vi "BMonitor.vi"   [LabVIEW 2016]
uses:
  Instrument_Setup.vi
  Global/Global Variables/Data_Display_global.vi
types:
  T1 = typedef "PSIO.ctl" = cluster{"Address":T2, "Version":enum16{"PS", "IPS"}}
  T2 = typedef "OxfordAddress.ctl" = cluster{"Com Port":i32, "ISOBUS Address":i32, "GPIB Address":i16, "Communication":enum16{"RS232", "ISOBUS", "GPIB", "Gateway"}}
  T3 = cluster{"Value":i16, "At rest":bool, "Sweeping":bool, "Rate limiting":bool}
  T4 = cluster{"Value":i16, "Hold":bool, "To set point":bool, "To zero":bool, "Clamped":bool}
  T5 = cluster{"Value":i16, "Off (at zero field)":bool, "On":bool, "Off (at field)":bool, "No switch fitted":bool, "Confirm":bool}
  T6 = cluster{"Value":i16, "Desired":u16, "Magnet":u16, "Commanded":u16, "Actual":u16}
  T7 = cluster{"Value":i16, "Quenched":bool, "Over heated":bool, "Warming up":bool}
  T8 = cluster{"Clamp":bool, "Settings":bool, "Switch Heater":bool, "Go to Zero":bool, "Go to set\nGo to Set":bool, "Go to Hold":bool, "Clamped":bool, "Quenched":bool, "Rate limit":bool, "Persistent":bool, "Hold":bool, "Set":bool, "Zero":bool, "Magnet (T)":dbl, "Leads (T)":dbl, "Magnet T (K)":dbl, "Confirm":bool, "Select":bool}
  T9 = typedef "PSSetupArray.ctl" = T10[]
  T10 = typedef "PSSetup.ctl" = cluster{"Max Sweep(4.2K)":dbl[unit], "Max Sweep(2.2K)":dbl[unit], "Switch htr dly":dbl[unit], "O/P contactor?":bool, "Max Field(4.2K)":dbl[unit], "Max Field(2.2K)":dbl[unit], "Description\n":string, "Settings.vi":path, "Max lead res":dbl[unit], "IO Info":T1, "Adjust shims":bool}
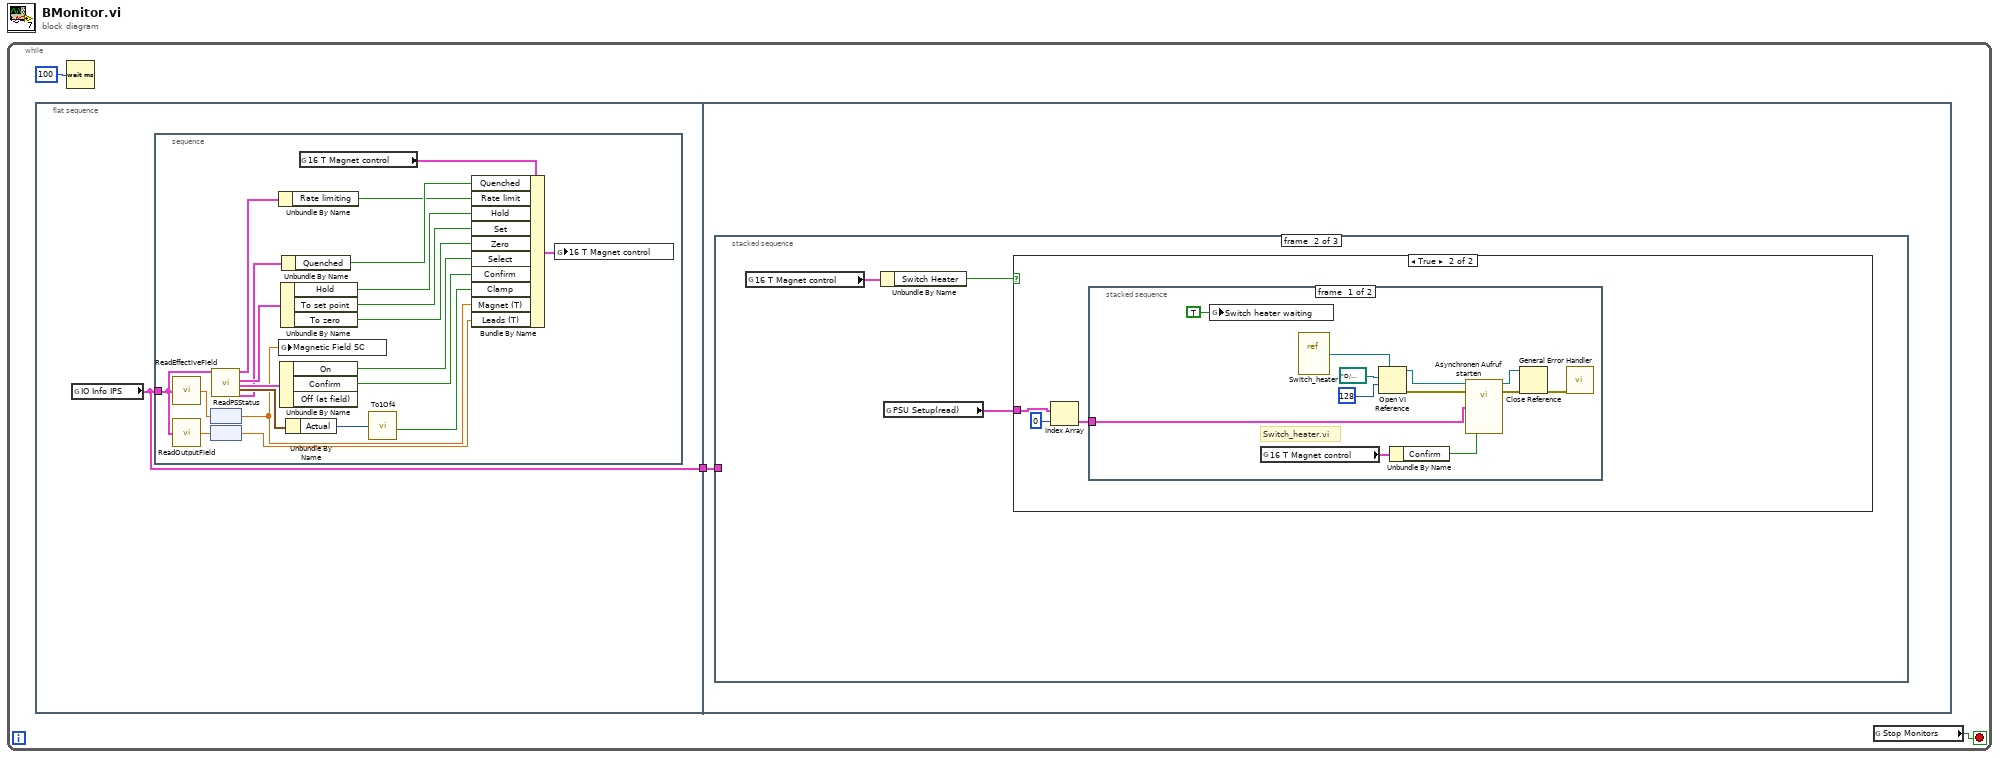
[diagram p0: block diagram]
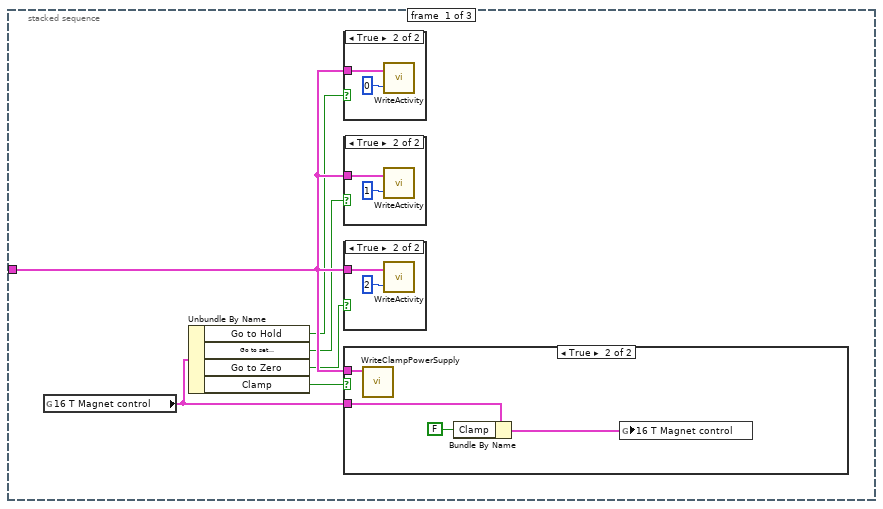
[diagram p2: hidden frame]
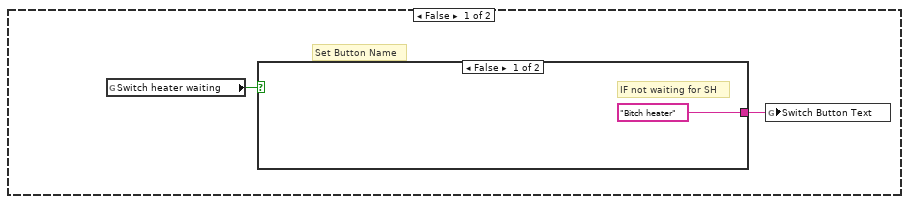
[diagram p7: hidden frame]
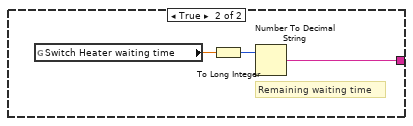
[diagram p8: hidden frame]
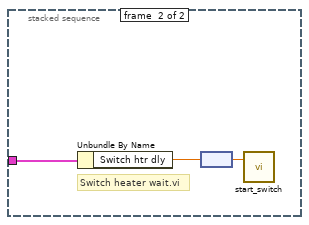
[diagram p9: hidden frame]
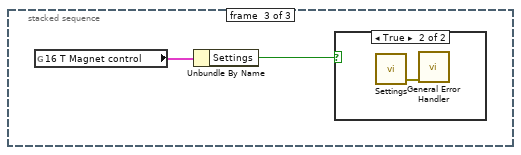
[diagram p10: hidden frame]
diagram:
  n1 = while {
    stop <- w3 stop-if-true
    n2 = flat-sequence {
      tunnel: [w4] -> w1
      tunnel: w1 -> [w26]
      frame #0 {
        n3 = global read "Instrument_Setup.vi" "IO Info IPS"() -> (w4:T1)
        n4 = stacked-sequence {
          tunnel: w4 -> [w7]
          frame #0 {
            n5 = call "ReadEffectiveField.vi"("IO Info"=w7) -> ("Effective field"=w6:dbl[unit])  [unwired: 2 out]
            n6 = call "ReadOutputField.vi"("IO Info"=w7) -> ("Field"=w9:dbl[unit])  [unwired: 2 out]
            n7 = node(w6) -> (w5:dbl)
            n8 = node(w9) -> (w8:dbl)
            n9 = call "ReadPSStatus.vi"("IO Info"=w7) -> ("Mode (n)"=w23:T3, "Activity"=w24:T4, "Switch Heater"=w22:T5, "Polarity"=w21:T6, "System Status (m)"=w20:T7)  [unwired: 10 in, 4 out]
            n10 = Unbundle By Name(w23) -> ("Rate limiting"=w15:bool)
            n11 = global write "Data_Display_global.vi" "Magnetic Field SC"(w5) -> ()
            n12 = Unbundle By Name(w22) -> ("On"=w11:bool, "Confirm"=w10:bool)  [unwired: 1 out]
            n13 = Unbundle By Name(w24) -> ("Hold"=w14:bool, "To set point"=w13:bool, "To zero"=w12:bool)
            n14 = Unbundle By Name(w20) -> ("Quenched"=w16:bool)
            n15 = Unbundle By Name(w21) -> ("Actual"=w25:u16)
            n16 = global read "Data_Display_global.vi" "16 T Magnet control"() -> (w19:T8)
            n17 = call "To1Of4.vi"("Input"=w25) -> ("3"=w17:bool)  [unwired: 3 out]
            n18 = Bundle By Name(cluster=w19, "Quenched"=w16, "Rate limit"=w15, "Hold"=w14, "Set"=w13, "Zero"=w12, "Select"=w11, "Confirm"=w10, "Clamp"=w17, "Magnet (T)"=w5, "Leads (T)"=w8) -> (w18:T8)
            n19 = global write "Data_Display_global.vi" "16 T Magnet control"(w18) -> ()
          }
        }
      }
      frame #1 {
        n20 = stacked-sequence {
          tunnel: w26 -> [w32 _ _]
          frame #0 {
            n21 = global read "Data_Display_global.vi" "16 T Magnet control"() -> (w27:T8)
            n22 = Unbundle By Name(w27) -> ("Go to Hold"=w31:bool, "Go to set\nGo to Set"=w30:bool, "Go to Zero"=w29:bool, "Clamp"=w28:bool)
            n23 = case shown="True" w31 {
              tunnel: w32 -> [_ w42]
              frame False {
              }
              frame True {
                n24 = call "WriteActivity.vi"("Activity"=0, "IO Info"=w42) -> ()  [unwired: 1 in, 1 out]
              }
            }
            n25 = case shown="True" w30 {
              tunnel: w32 -> [_ w40]
              frame False {
              }
              frame True {
                n26 = call "WriteActivity.vi"("Activity"=1, "IO Info"=w40) -> ()  [unwired: 1 in, 1 out]
              }
            }
            n27 = case shown="True" w29 {
              tunnel: w32 -> [_ w38]
              frame False {
              }
              frame True {
                n28 = call "WriteActivity.vi"("Activity"=2, "IO Info"=w38) -> ()  [unwired: 1 in, 1 out]
              }
            }
            n29 = case shown="True" w28 {
              tunnel: w32 -> [_ w36]
              tunnel: w27 -> [_ w34]
              frame False {
              }
              frame True {
                n30 = call "WriteClampPowerSupply.vi"("IO Info"=w36) -> ()  [unwired: 9 in, 2 out]
                n31 = Bundle By Name(cluster=w34, "Clamp"=FALSE) -> (w33:T8)
                n32 = global write "Data_Display_global.vi" "16 T Magnet control"(w33) -> ()
              }
            }
          }
          frame #1 {
            n33 = global read "Data_Display_global.vi" "16 T Magnet control"() -> (w45:T8)
            n34 = Unbundle By Name(w45) -> ("Switch Heater"=w44:bool)
            n35 = global read "Instrument_Setup.vi" "PSU Setup(read)"() -> (w43:T9)
            n36 = case shown="True" w44 {
              tunnel: w43 -> [_ w54]
              frame False {
                # "Set Button Name"
                n37 = global read "Data_Display_global.vi" "Switch heater waiting"() -> (w47:bool)
                n38 = case shown="False" w47 {
                  tunnel: ["Bitch heater" w49] -> w46
                  frame False {
                    # "IF not waiting for SH"
                  }
                  frame True {
                    # "Remaining waiting time"
                    n39 = global read "Data_Display_global.vi" "Switch Heater waiting time"() -> (w51:dbl)
                    n40 = To Long Integer(number=w51) -> (32bit integer=w50:i32)
                    n41 = Number To Decimal String(number=w50) -> (decimal integer string=w49:string)  [unwired: 1 in]
                  }
                }
                n42 = global write "Data_Display_global.vi" "Switch Button Text"(w46) -> ()
              }
              frame True {
                n43 = Index Array(array=w54, index=0) -> (element=w52:T10)
                n44 = stacked-sequence {
                  tunnel: w52 -> [w55 w67]
                  frame #0 {
                    # "Switch_heater.vi"
                    n45 = global write "Data_Display_global.vi" "Switch heater waiting"(TRUE) -> ()
                    n46 = global read "Data_Display_global.vi" "16 T Magnet control"() -> (w57:T8)
                    n47 = vi-ref "Switch_heater.vi"() -> (w66:refnum<vi>)
                    n48 = Open VI Reference(type specifier VI Refnum (for type only)=w66, vi path=path "D:/Cryostat Software/CryoTUM-V1.0/sub_vi-s/Equipment/ITC/Switch_heater.vi" ("VI-Pfad"), options=128) -> (vi reference=w65:refnum<vi>, error out=w63:errorcluster)  [unwired: 3 in]
                    n49 = Unbundle By Name(w57) -> ("Confirm"=w56:bool)
                    n50 = call-by-ref "Asynchronen Aufruf starten"(reference=w65, error in=w63, "Boolesch"=w56, "PSU Setup"=w55) -> (reference out=w59:refnum<vi>, error out=w60:errorcluster)  [unwired: 2 in]
                    n51 = Close Reference(reference=w59, error in (no error)=w60) -> (error out=w64:errorcluster)
                    n52 = call <vilib>:"General Error Handler.vi"("error in (no error)"=w64) -> ()  [unwired: 10 in, 5 out]
                  }
                  frame #1 {
                    # "Switch heater wait.vi"
                    n53 = Unbundle By Name(w67) -> ("Switch htr dly"=w69:dbl[unit])
                    n54 = node(w69) -> (w68:dbl)
                    n55 = call "start_switch.vi"("Switch heater time"=w68) -> ()  [unwired: 2 in]
                  }
                }
              }
            }
          }
          frame #2 {
            n56 = global read "Data_Display_global.vi" "16 T Magnet control"() -> (w70:T8)
            n57 = Unbundle By Name(w70) -> ("Settings"=w71:bool)
            n58 = case shown="True" w71 {
              frame False {
              }
              frame True {
                n59 = call "Settings.vi"() -> ("error out"=w72:errorcluster)  [unwired: 5 in]
                n60 = call <vilib>:"General Error Handler.vi"("error in (no error)"=w72) -> ()  [unwired: 10 in, 5 out]
              }
            }
          }
        }
      }
    }
    n61 = Wait (ms)(milliseconds to wait=100) -> ()  [unwired: 1 out]
    n62 = global read "Data_Display_global.vi" "Stop Monitors"() -> (w3:bool)
  }
